vi "ST4H.vi"(10 "STOIL_path":path=path "C:/Users/lsv/Documents/Sys/AI-04/air-speed/VI/STOIL.FOR", 11 "H":dbl) -> (2 "T":dbl, 3 "S":dbl)   [LabVIEW 2020]
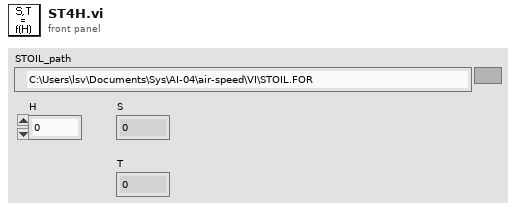
[diagram p1: front panel]
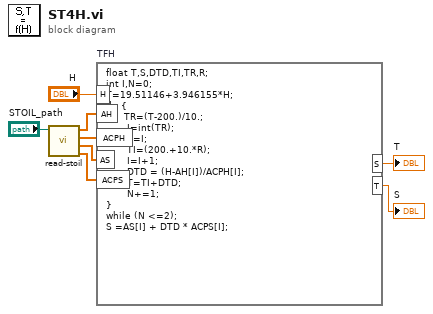
[diagram p0: block diagram]
diagram:
  n1 = call "read-stoil.vi"("file path (use dialog)"="STOIL_path") -> ("ACPS"=w4:dbl[], "AS"=w3:dbl[], "ACPH"=w5:dbl[], "AH"=w6:dbl[])  [unwired: 7 in]
  n2 = formula code="float T,S,DTD,TI,TR,R;\nint I,N=0;\nT=19.51146+3.946155*H;\ndo {\n      TR=(T-200.)/10.;\n       I=int(TR);\n       R=I;\n       TI=(200.+10.*R);\n       I=I+1;\n       DTD = (H-AH[I])/ACPH[I];\n       T=TI+DTD;\n       N+=1;\n}\nwhile (N <=2);\nS =AS[I] + DTD * ACPS[I];" "TFH"("H"="H", "AS"=w3, "ACPS"=w4, "AH"=w6, "ACPH"=w5) -> ("T"=→"S":dbl, "S"=→"T":dbl)
